vi "Actor Core.vi"(8 "error in":errorcluster, 11 "File Provider in":refnum<class "File Provider.lvclass">) -> (0 "error out":errorcluster, 3 "Actor out":refnum<class "Actor.lvclass">)   [LabVIEW 2023, in "File Provider.lvlib" / "File Provider.lvclass"]
doc: "(<B>Filename</B>: Actor Framework.lvlib:Actor.lvclass:Actor Core.vi)\n\nReceives messages to the actor, reacts to them, and initiates any error handling that may shut the actor down.\n\nDescendant classes may override this VI to append parallel tasks for the actor to complete while it handles messages. Overrides use the Call Parent Class Method node."
uses:
  File Provider.lvclass
  File Provider.lvclass/File Provider.ctl
  <vilib>/MGI/Panel Manager/Panel Actor/Panel Actor/Panel Actor.lvclass
  <vilib>/ActorFramework/Actor/Actor.lvclass
panel:
  in  "Load Button":bool
  out "Instr CFGs":string[](array[string])
  in  "Series Instr CFG":path
  in  "Virt Instr CFG":path
  in  "Instr CFG":path
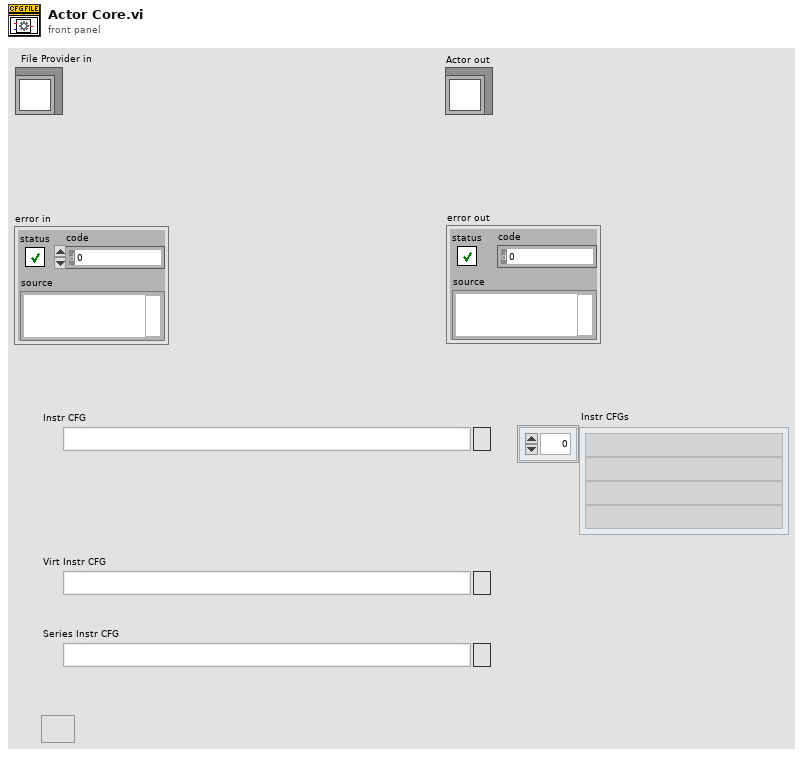
[diagram p1: front panel]
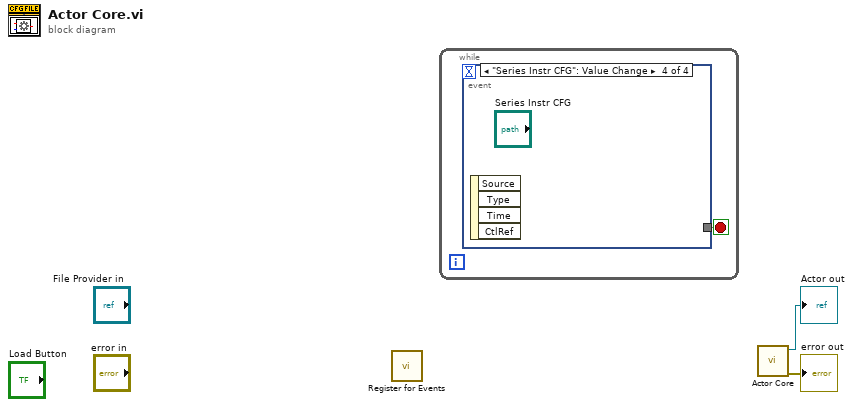
[diagram p0: block diagram]
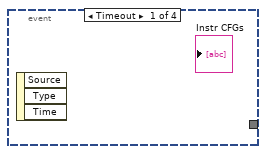
[diagram p2: hidden frame]
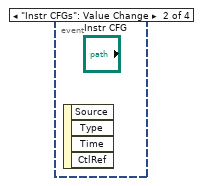
[diagram p3: hidden frame]
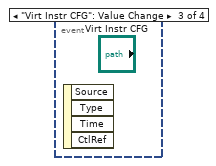
[diagram p4: hidden frame]
diagram:
  n1 = call <vilib>:"Register for Events.vi"() -> ()  [unwired: 8 in, 4 out]
  n2 = while {
    stop <- w4 stop-if-true
    n3 = event shown="[3] \"Series Instr CFG\": Value Change" {
      selector: _ -> [_ _ _ _]
      dyn-events: _ -> [_ _ _ _]
      timeout: _ -> [_ _ _ _]
      tunnel: [_ _ _ _] -> w4
      event Timeout {
        n4 = event-data() -> ()  [unwired: 1 in, 3 out]
      }
      event "Instr CFGs": Value Change {
        n5 = event-data() -> ()  [unwired: 1 in, 4 out]
      }
      event "Virt Instr CFG": Value Change {
        n6 = event-data() -> ()  [unwired: 1 in, 4 out]
      }
      event "Series Instr CFG": Value Change {
        n7 = event-data() -> ()  [unwired: 1 in, 4 out]
      }
    }
  }
  n8 = call-parent "Actor Core.vi"() -> ("error out"=→"error out":errorcluster, "Actor out"=→"Actor out":refnum<class "Actor.lvclass">, "Actor in"=w1:refnum<class "File Provider.lvclass">)  [unwired: 9 in]
